vi "Limits1.vi"() -> ()   [LabVIEW 2019]
uses:
  Supported.llb/Global-1.vi
panel:
  out "upper limit":dbl
  out "lower limit":dbl
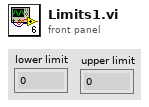
[diagram p1: front panel]
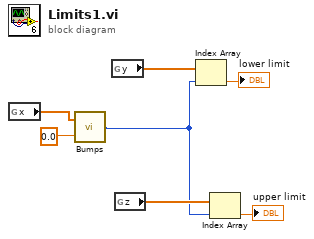
[diagram p0: block diagram]
diagram:
  n1 = global read "Global-1.vi" "x"() -> (w1:dbl[])
  n2 = call "Bumps.vi"("lower limit"=0.0, "Array in"=w1) -> ("Index out"=w3:i32)
  n3 = global read "Global-1.vi" "y"() -> (w7:dbl[])
  n4 = global read "Global-1.vi" "z"() -> (w4:dbl[])
  n5 = Index Array(array=w7, index=w3) -> (element=→"lower limit":dbl)
  n6 = Index Array(array=w4, index=w3) -> (element=→"upper limit":dbl)
